vi "Parse.vi"(8 "Error In":errorcluster, 11 "object in":refnum<class "2022_3.lvclass">) -> (0 "Error Out":errorcluster, 3 "object out":refnum<class "2022_3.lvclass">)   [LabVIEW 2023, in "2022_3.lvclass"]
uses:
  2022_3.lvclass
  2022_3.lvclass/2022_3.ctl
  <vilib>/Utility/error.llb/Trim Whitespace One-Sided.vi
  <userlib>/_OpenG.lib/string/string.llb/openg_string.lvlib
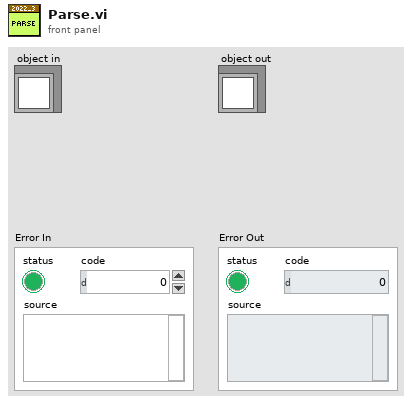
[diagram p1: front panel]
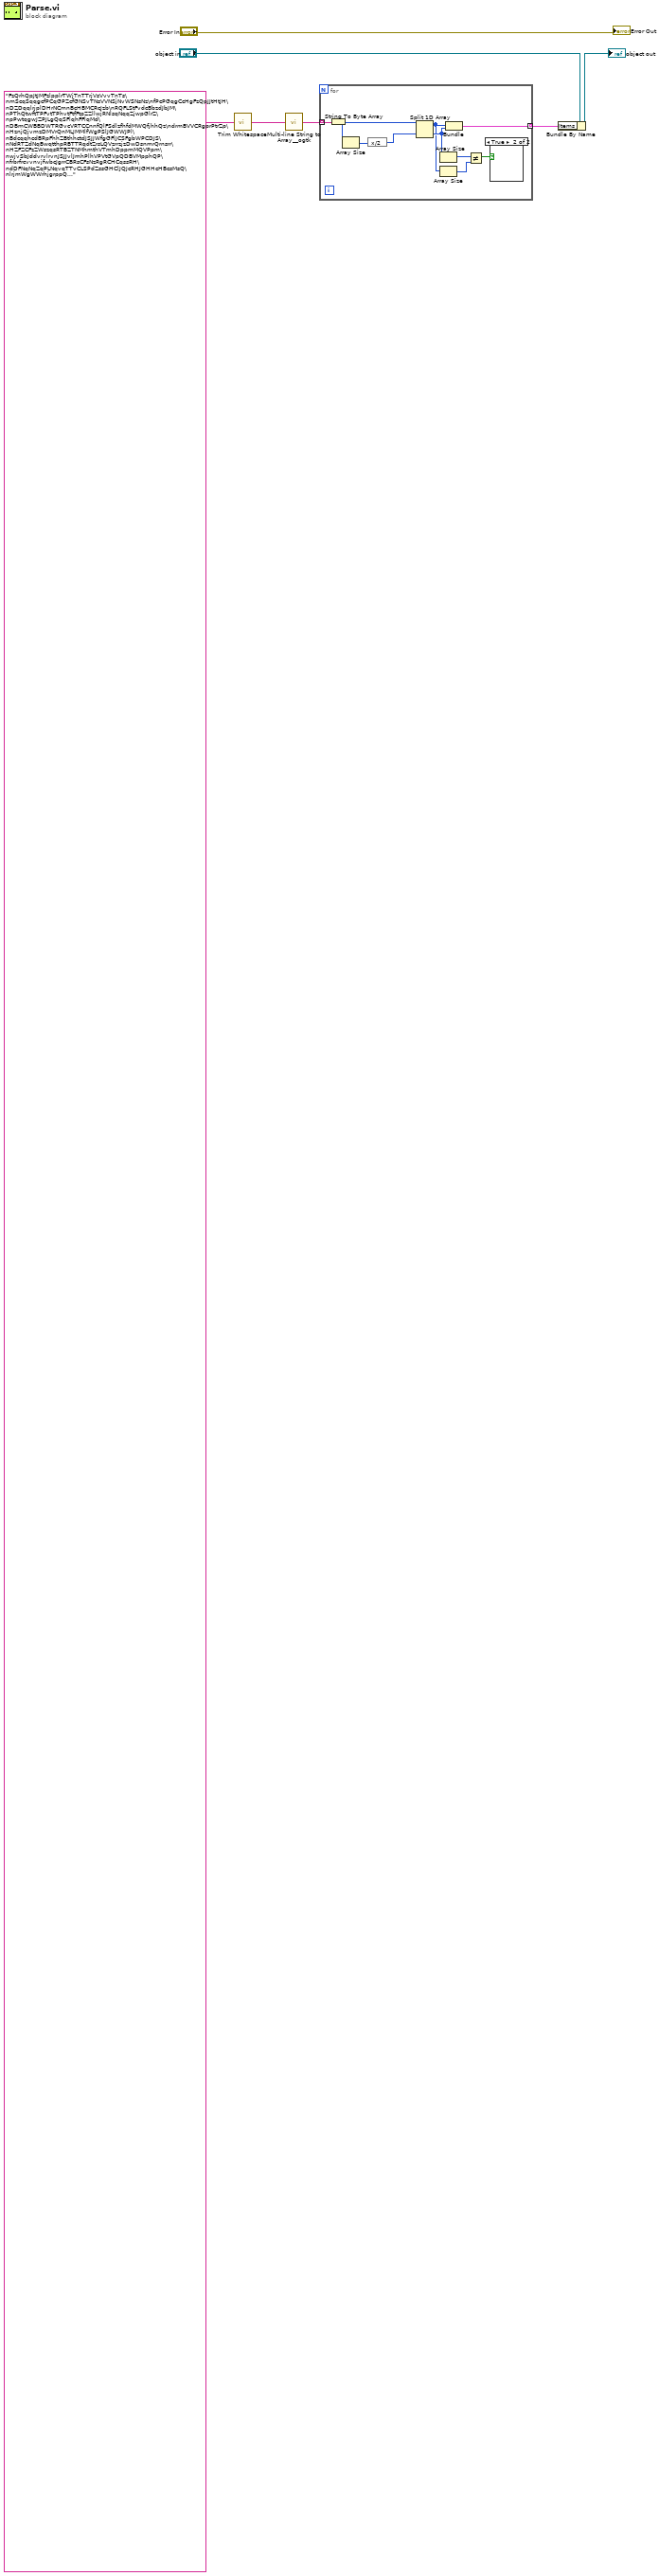
[diagram p0: block diagram]
diagram:
  n1 = call <vilib>:"Trim Whitespace.vi"("string"="FzQrhQpJtJMFzlpplrTWjTnTTrjVsVvvTnTs\nmScqSqqgcfPCqGPZcfGNSvTNsVVNSjNvWSNsNz\nfPcPGqgCcHgFzQpJJtHtJH\nDZDqqlrjplDHrNCmnBcHBMCRcJzb\nRQFLStFvdcBbzdJbJM\nPThQtwftTPFvtTPhvtFtfFtpZZllwjRNlsqNqqZjwpGlrZ\npPwtqgwJZPJLgQqSFlqhFFlqMd\nDBmCWBBDWTRGvcVRTCCnnfQlFSdlzfhfdMWQfjhhQz\ndrmBVVCRgprPtrZp\nHznjQjvmzDMVrQnMLJMMlfWgPSlJGWWJPl\nBdcqqhcdBRpFhhZBthhctdJSJJWfgGFlJCSFgbWPCDJS\nNdRTZdNqBwqtthpRBTTRqdtZrsLQVzrrzjzDwDsnmrQrnsrr\nHZFZCFzZWszqsRTBZTNMhmthVTmhDppmMQVPpm\nwjvSbJddvrvlrvnJSJJvlJmhPlhVPVtGVpQDBVMpphQP\nfrbrfrcvvnvjfwbcJgrrCBRsCFsNzRgRCHCqssRH\ndDFNqNqZqPLNqvqTTvCLSPdZssGHClJQJcRHJGHHcHBcsMsQ\nlrjmWgWWrhjgrppQ..." ("PuzzleInput")) -> ("trimmed string"=w3:string)  [unwired: 1 in]
  n2 = call <userlib>:"Multi-line String to Array__ogtk.vi"("string"=w3) -> ("lines"=w2:string[])
  n3 = for {
    tunnel: w2 -> [w17] mode=indexing
    tunnel: [w13] -> w1 mode=indexing
    n4 = String To Byte Array(string=w17) -> (unsigned byte array=w16:u8[])
    n5 = Array Size(array=w16) -> (size(s)=w15:i32)
    n6 = expression code="x/2"(w15) -> (w14:i32)
    n7 = Split 1D Array(array=w16, index=w14) -> (first subarray=w11:u8[], second subarray=w12:u8[])
    n8 = Array Size(array=w12) -> (size(s)=w10:i32)
    n9 = Array Size(array=w11) -> (size(s)=w9:i32)
    n10 = Bundle(w11, w12) -> (w13:cluster{u8[], u8[]})  [unwired: 1 in]
    n11 = Not Equal?(x=w10, y=w9) -> (x != y?=w8:bool)
    n12 = case shown="True" w8 {
      frame False {
      }
      frame True {
      }
    }
  }
  n13 = Bundle By Name(cluster="object in", "Items"=w1) -> (→"object out":refnum<class "2022_3.lvclass">)
  "Error Out" <- "Error In"
